vi "Variant Constant (array).vi"() -> (1 "array":variant[](array[variant]))   [LabVIEW 2015]
doc: "Empty variant (void variant wrapped by variant) represents null on serialization."
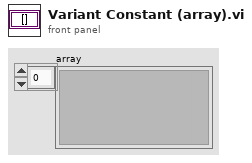
[diagram p1: front panel]
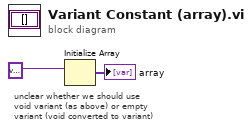
[diagram p0: block diagram]
diagram:
  # "unclear whether we should use\nvoid variant (as above) or empty\nvariant (void converted to variant)"
  n1 = Initialize Array(variant) -> (→"array":variant[])  [unwired: 1 in]
